vi "Creat file for Seq path.vi"(11 "ini in":T4) -> (3 "Paths of Sequence":T1)   [LabVIEW 2018]
uses:
  type defs/Sequence paths.ctl
  type defs/Sequence Info.ctl
  type defs/Sequence Status.ctl
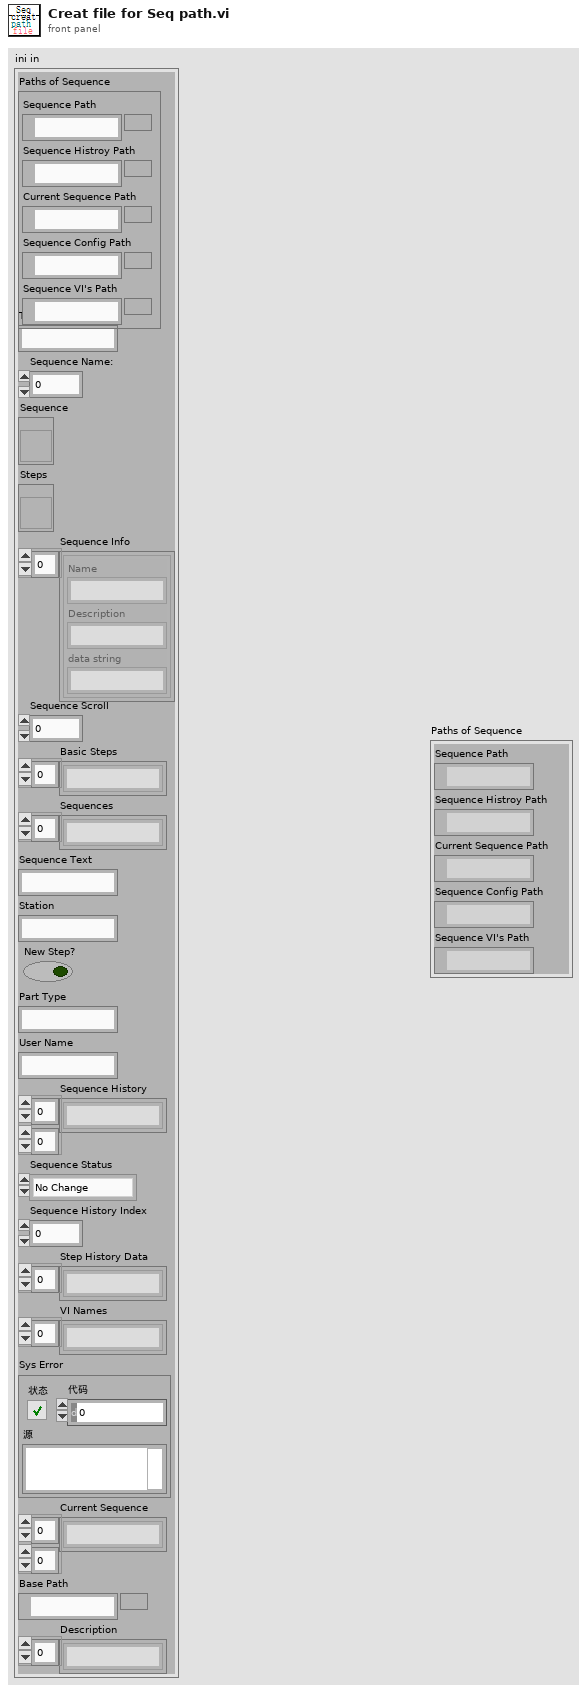
[diagram p1: front panel]
types:
  T1 = typedef "Sequence paths.ctl" = cluster{"Sequence Path":path, "Sequence Histroy Path":path, "Current Sequence Path":path, "Sequence Config Path":path, "Sequence VI's Path":path}
  T2 = typedef "Sequence Info.ctl" = cluster{"Name":string, "Description":string, "data string":string}
  T3 = typedef "Sequence Status.ctl" = enum16{"No Change", "Edited", "New Step", "Deleted", "Moved Up", "Moved Down", "Copied"}
  T4 = cluster{"Paths of Sequence":T1, "Type":string, "Sequence Name:":i32, "Sequence":refnum<vi>, "Steps":refnum<vi>, "Sequence Info":T2[], "Sequence Scroll":u32, "Basic Steps":string[], "Sequences":string[], "Sequence Text":string, "Station":string, "New Step?":bool, "Part Type":string, "User Name":string, "Sequence History":string[][], "Sequence Status":T3, "Sequence History Index":i32, "Step History Data":string[], "VI Names":string[], "Sys Error":errorcluster, "Current Sequence":string[][], "Base Path":path, "Description":string[]}
  T5 = enum16{"open", "replace", "create", "open or create", "replace or create", "replace or create with confirmation"}
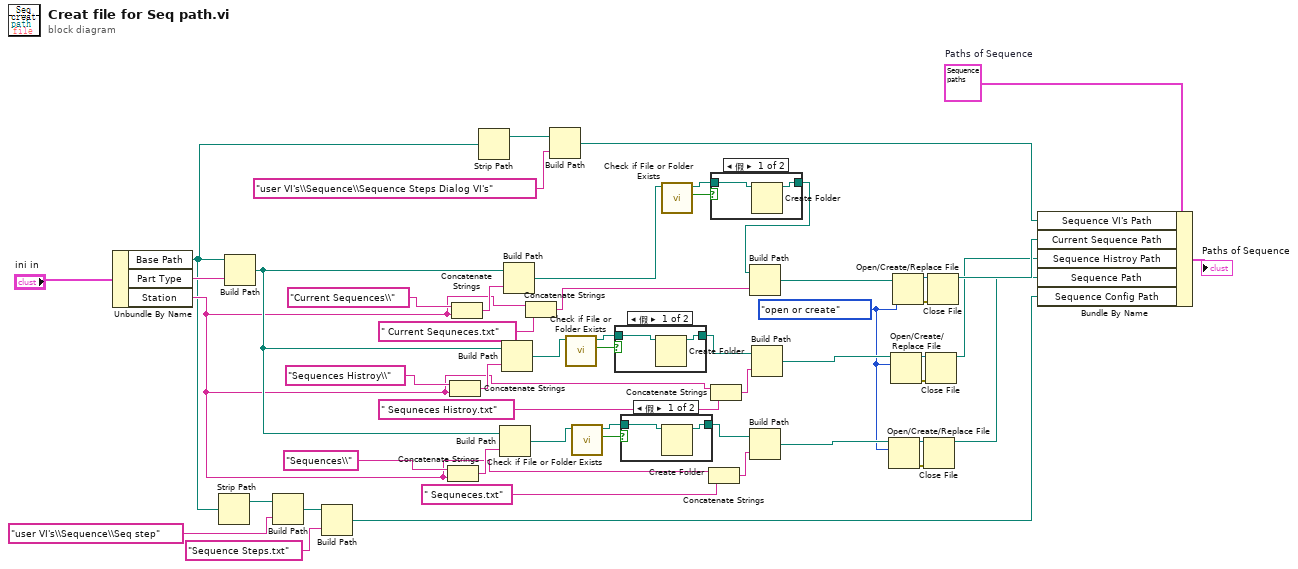
[diagram p0: block diagram]
diagram:
  w15 = T1 {"Sequence Path"=path "", "Sequence Histroy Path"=path "", "Current Sequence Path"=path "", "Sequence Config Path"=path "", "Sequence VI's Path"=path ""}  # Paths of Sequence
  w30 = T5."open or create" ("操作(0:open)")
  n1 = Unbundle By Name("ini in") -> ("Base Path"=w4:path, "Part Type"=w52:string, "Station"=w10:string)
  n2 = Strip Path(path=w4) -> (stripped path=w3:path)  [unwired: 1 out]
  n3 = Build Path(base path=w4, name or relative path=w52) -> (appended path=w31:path)
  n4 = Build Path(base path=w3, name or relative path="user VI's\\Sequence\\Seq step" ("名称或相对路径")) -> (appended path=w1:path)
  n5 = Build Path(base path=w1, name or relative path="Sequence Steps.txt" ("名称或相对路径")) -> (appended path=w11:path)
  n6 = Concatenate Strings("Sequences\\", w10) -> (w36:string)
  n7 = Concatenate Strings("Sequences Histroy\\", w10) -> (w43:string)
  n8 = Concatenate Strings("Current Sequences\\", w10) -> (w49:string)
  n9 = Strip Path(path=w4) -> (stripped path=w7:path)  [unwired: 1 out]
  n10 = Build Path(base path=w31, name or relative path=w36) -> (appended path=w17:path)
  n11 = Build Path(base path=w31, name or relative path=w43) -> (appended path=w21:path)
  n12 = Build Path(base path=w31, name or relative path=w49) -> (appended path=w25:path)
  n13 = Concatenate Strings(w10, " Current Sequneces.txt" ("字符串")) -> (w50:string)
  n14 = Build Path(base path=w7, name or relative path="user VI's\\Sequence\\Sequence Steps Dialog VI's" ("名称或相对路径")) -> (appended path=w5:path)
  n15 = call <vilib>:"Check if File or Folder Exists.vi"("path"=w21) -> ("file or folder exists?"=w23:bool, "dup path"=w22:path)  [unwired: 8 in, 1 out]
  n16 = call <vilib>:"Check if File or Folder Exists.vi"("path"=w17) -> ("file or folder exists?"=w19:bool, "dup path"=w18:path)  [unwired: 8 in, 1 out]
  n17 = case shown="假" w23 {
    tunnel: [w53 w55] -> w20
    tunnel: w22 -> [w54 w55]
    frame False {
      n18 = Create Folder(path (use dialog)=w54) -> (created path=w53:path)  [unwired: 2 in, 2 out]
    }
    frame True {
    }
  }
  n19 = case shown="假" w19 {
    tunnel: [w56 w58] -> w16
    tunnel: w18 -> [w57 w58]
    frame False {
      n20 = Create Folder(path (use dialog)=w57) -> (created path=w56:path)  [unwired: 2 in, 2 out]
    }
    frame True {
    }
  }
  n21 = call <vilib>:"Check if File or Folder Exists.vi"("path"=w25) -> ("file or folder exists?"=w28:bool, "dup path"=w27:path)  [unwired: 8 in, 1 out]
  n22 = Concatenate Strings(w10, " Sequneces.txt" ("字符串")) -> (w37:string)
  n23 = case shown="假" w28 {
    tunnel: [w59 w61] -> w24
    tunnel: w27 -> [w60 w61]
    frame False {
      n24 = Create Folder(path (use dialog)=w60) -> (created path=w59:path)  [unwired: 2 in, 2 out]
    }
    frame True {
    }
  }
  n25 = Concatenate Strings(w10, " Sequneces Histroy.txt" ("字符串")) -> (w44:string)
  n26 = Build Path(base path=w24, name or relative path=w50) -> (appended path=w26:path)
  n27 = Build Path(base path=w16, name or relative path=w37) -> (appended path=w34:path)
  n28 = Build Path(base path=w20, name or relative path=w44) -> (appended path=w41:path)
  n29 = Open/Create/Replace File(file path (use dialog)=w34, operation (0:open)=w30) -> (refnum out=w32:refnum<file>, error out=w33:errorcluster)  [unwired: 4 in, 1 out]
  n30 = Open/Create/Replace File(file path (use dialog)=w41, operation (0:open)=w30) -> (refnum out=w39:refnum<file>, error out=w40:errorcluster)  [unwired: 4 in, 1 out]
  n31 = Open/Create/Replace File(file path (use dialog)=w26, operation (0:open)=w30) -> (refnum out=w46:refnum<file>, error out=w47:errorcluster)  [unwired: 4 in, 1 out]
  n32 = Close File(refnum=w32, error in=w33) -> (path=w12:path)  [unwired: 1 out]
  n33 = Close File(refnum=w39, error in=w40) -> (path=w13:path)  [unwired: 1 out]
  n34 = Close File(refnum=w46, error in=w47) -> (path=w14:path)  [unwired: 1 out]
  n35 = Bundle By Name(cluster=w15, "Sequence VI's Path"=w5, "Current Sequence Path"=w14, "Sequence Histroy Path"=w13, "Sequence Path"=w12, "Sequence Config Path"=w11) -> (→"Paths of Sequence":T1)
